vi "power command.vi"(1 "channel":T1, 2 "power [0-1022]":u16 max=1022 step=1) -> (0 "resulting string incl crc":string)   [LabVIEW 2018]
uses:
  chan select.ctl
panel:
  out "CRC":u8 format="%x"
  out "concatenated string":string
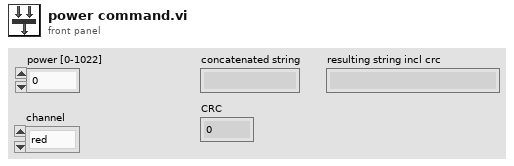
[diagram p1: front panel]
types:
  T1 = typedef "chan select.ctl" = enum16{"red", "green", "blue"}
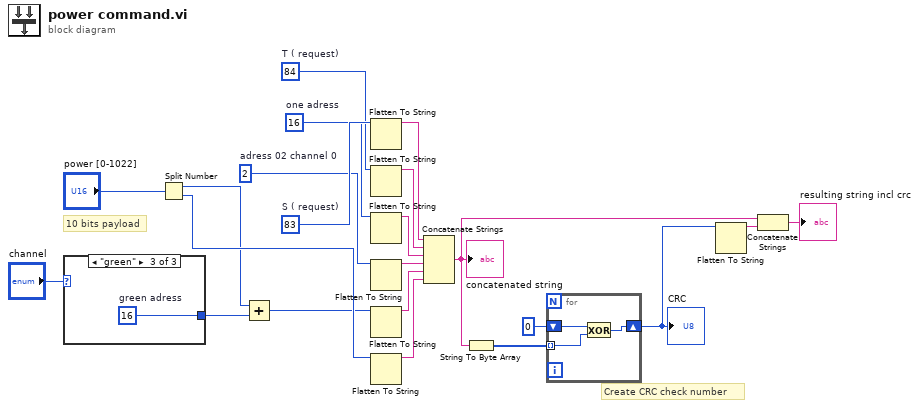
[diagram p0: block diagram]
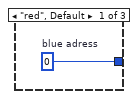
[diagram p2: hidden frame]
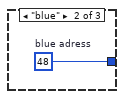
[diagram p3: hidden frame]
diagram:
  w14 = i8 2  # adress 02 channel 0
  w15 = i8 16  # one adress
  w20 = i8 84  # T ( request)
  w22 = i8 83  # S ( request)
  # "10 bits payload"
  # "Create CRC check number"
  n1 = case shown="\"green\"" "channel" {
    tunnel: [w23 w24 w25] -> w7
    frame "red", Default {
      w23 = i8 0  # blue adress
    }
    frame "blue" {
      w24 = i8 48  # blue adress
    }
    frame "green" {
      w25 = i8 16  # green adress
    }
  }
  n2 = Split Number(x="power [0-1022]") -> (hi(x)=w16:u8, lo(x)=w17:u8)
  n3 = Add(x=w16, y=w7) -> (x+y=w9:u8)
  n4 = Flatten To String(anything=w22) -> (data string=w21:string)  [unwired: 3 in, 2 out]
  n5 = Flatten To String(anything=w20) -> (data string=w19:string)  [unwired: 3 in, 2 out]
  n6 = Flatten To String(anything=w15) -> (data string=w13:string)  [unwired: 3 in, 2 out]
  n7 = Flatten To String(anything=w14) -> (data string=w12:string)  [unwired: 3 in, 2 out]
  n8 = Flatten To String(anything=w9) -> (data string=w11:string)  [unwired: 3 in, 2 out]
  n9 = Flatten To String(anything=w17) -> (data string=w10:string)  [unwired: 3 in, 2 out]
  n10 = Concatenate Strings(w21, w19, w13, w12, w11, w10) -> (w3:string)
  "concatenated string" <- w3
  n11 = String To Byte Array(string=w3) -> (unsigned byte array=w6:u8[])
  n12 = for {
    tunnel: w6 -> [w27] mode=indexing
    shift-right: [w26] -> w4
    shift-left: u8 0 -> [w28]
    n13 = Exclusive Or(1:w27, 2:w28) -> (0:w26:u8)
  }
  "CRC" <- w4
  n14 = Flatten To String(anything=w4) -> (data string=w2:string)  [unwired: 3 in, 2 out]
  n15 = Concatenate Strings(w3, w2) -> (→"resulting string incl crc":string)
